vi "Get INFO from ini FILE - AMSServer.vi"(0 "ini Name":string="AMSServer.ini", 5 "Application Directory (Default if blank)":path, 11 "Error In":errorcluster) -> (1 "Settings":T3, 4 "ini Path":path=path "C:/Users/CK/workspace/LabVIEW/Configuration File Test/MyEXE.ini", 8 "AMS Connection Information":T1={"Connection "="SQL Server 32bit HPEnvy", "Username"="admin", "Password"="admin123"}, 10 "Settings Boolean":T2, 12 "MessageQ":string, 15 "Error Out":errorcluster)   [LabVIEW 2013]
uses:
  Controls/Connection Information Cluster.ctl
  <vilib>/Utility/config.llb/Read Key (String).vi
  <vilib>/Utility/config.llb/Read Key (Boolean).vi
  <vilib>/Utility/config.llb/NI_LVConfig.lvlib
  <vilib>/Utility/config.llb/Write Key (I32).vi
panel:
  out "Application Directory":path=path "C:/Users/CK/workspace/LabVIEW/Configuration File Test"
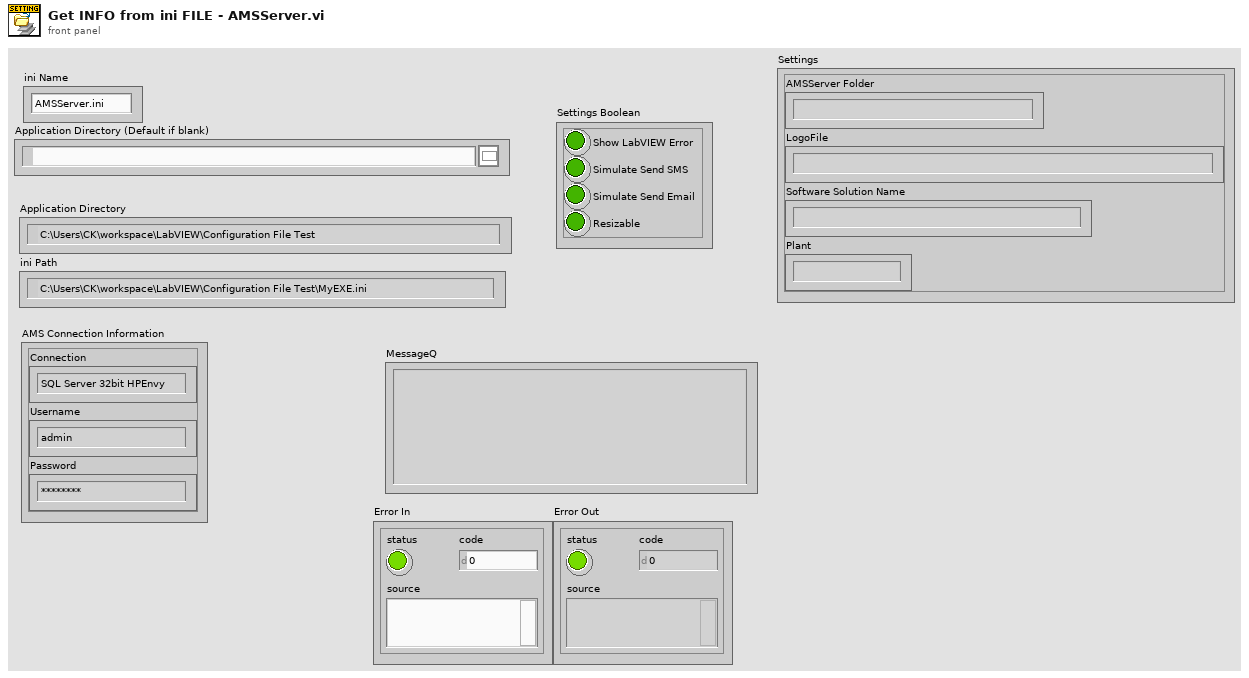
[diagram p1: front panel]
types:
  T1 = typedef "Connection Information Cluster.ctl" = cluster{"Connection ":string, "Username":string, "Password":string}
  T2 = cluster{"Show LabVIEW Error":bool, "Simulate Send SMS":bool, "Simulate Send Email":bool, "Resizable":bool}
  T3 = cluster{"AMSServer Folder":string, "LogoFile":string, "Software Solution Name":string, "Plant":string}
  T4 = typedef "NI_LVConfig.lvlib/Config Data RefNum.ctl" = refnum<k1>
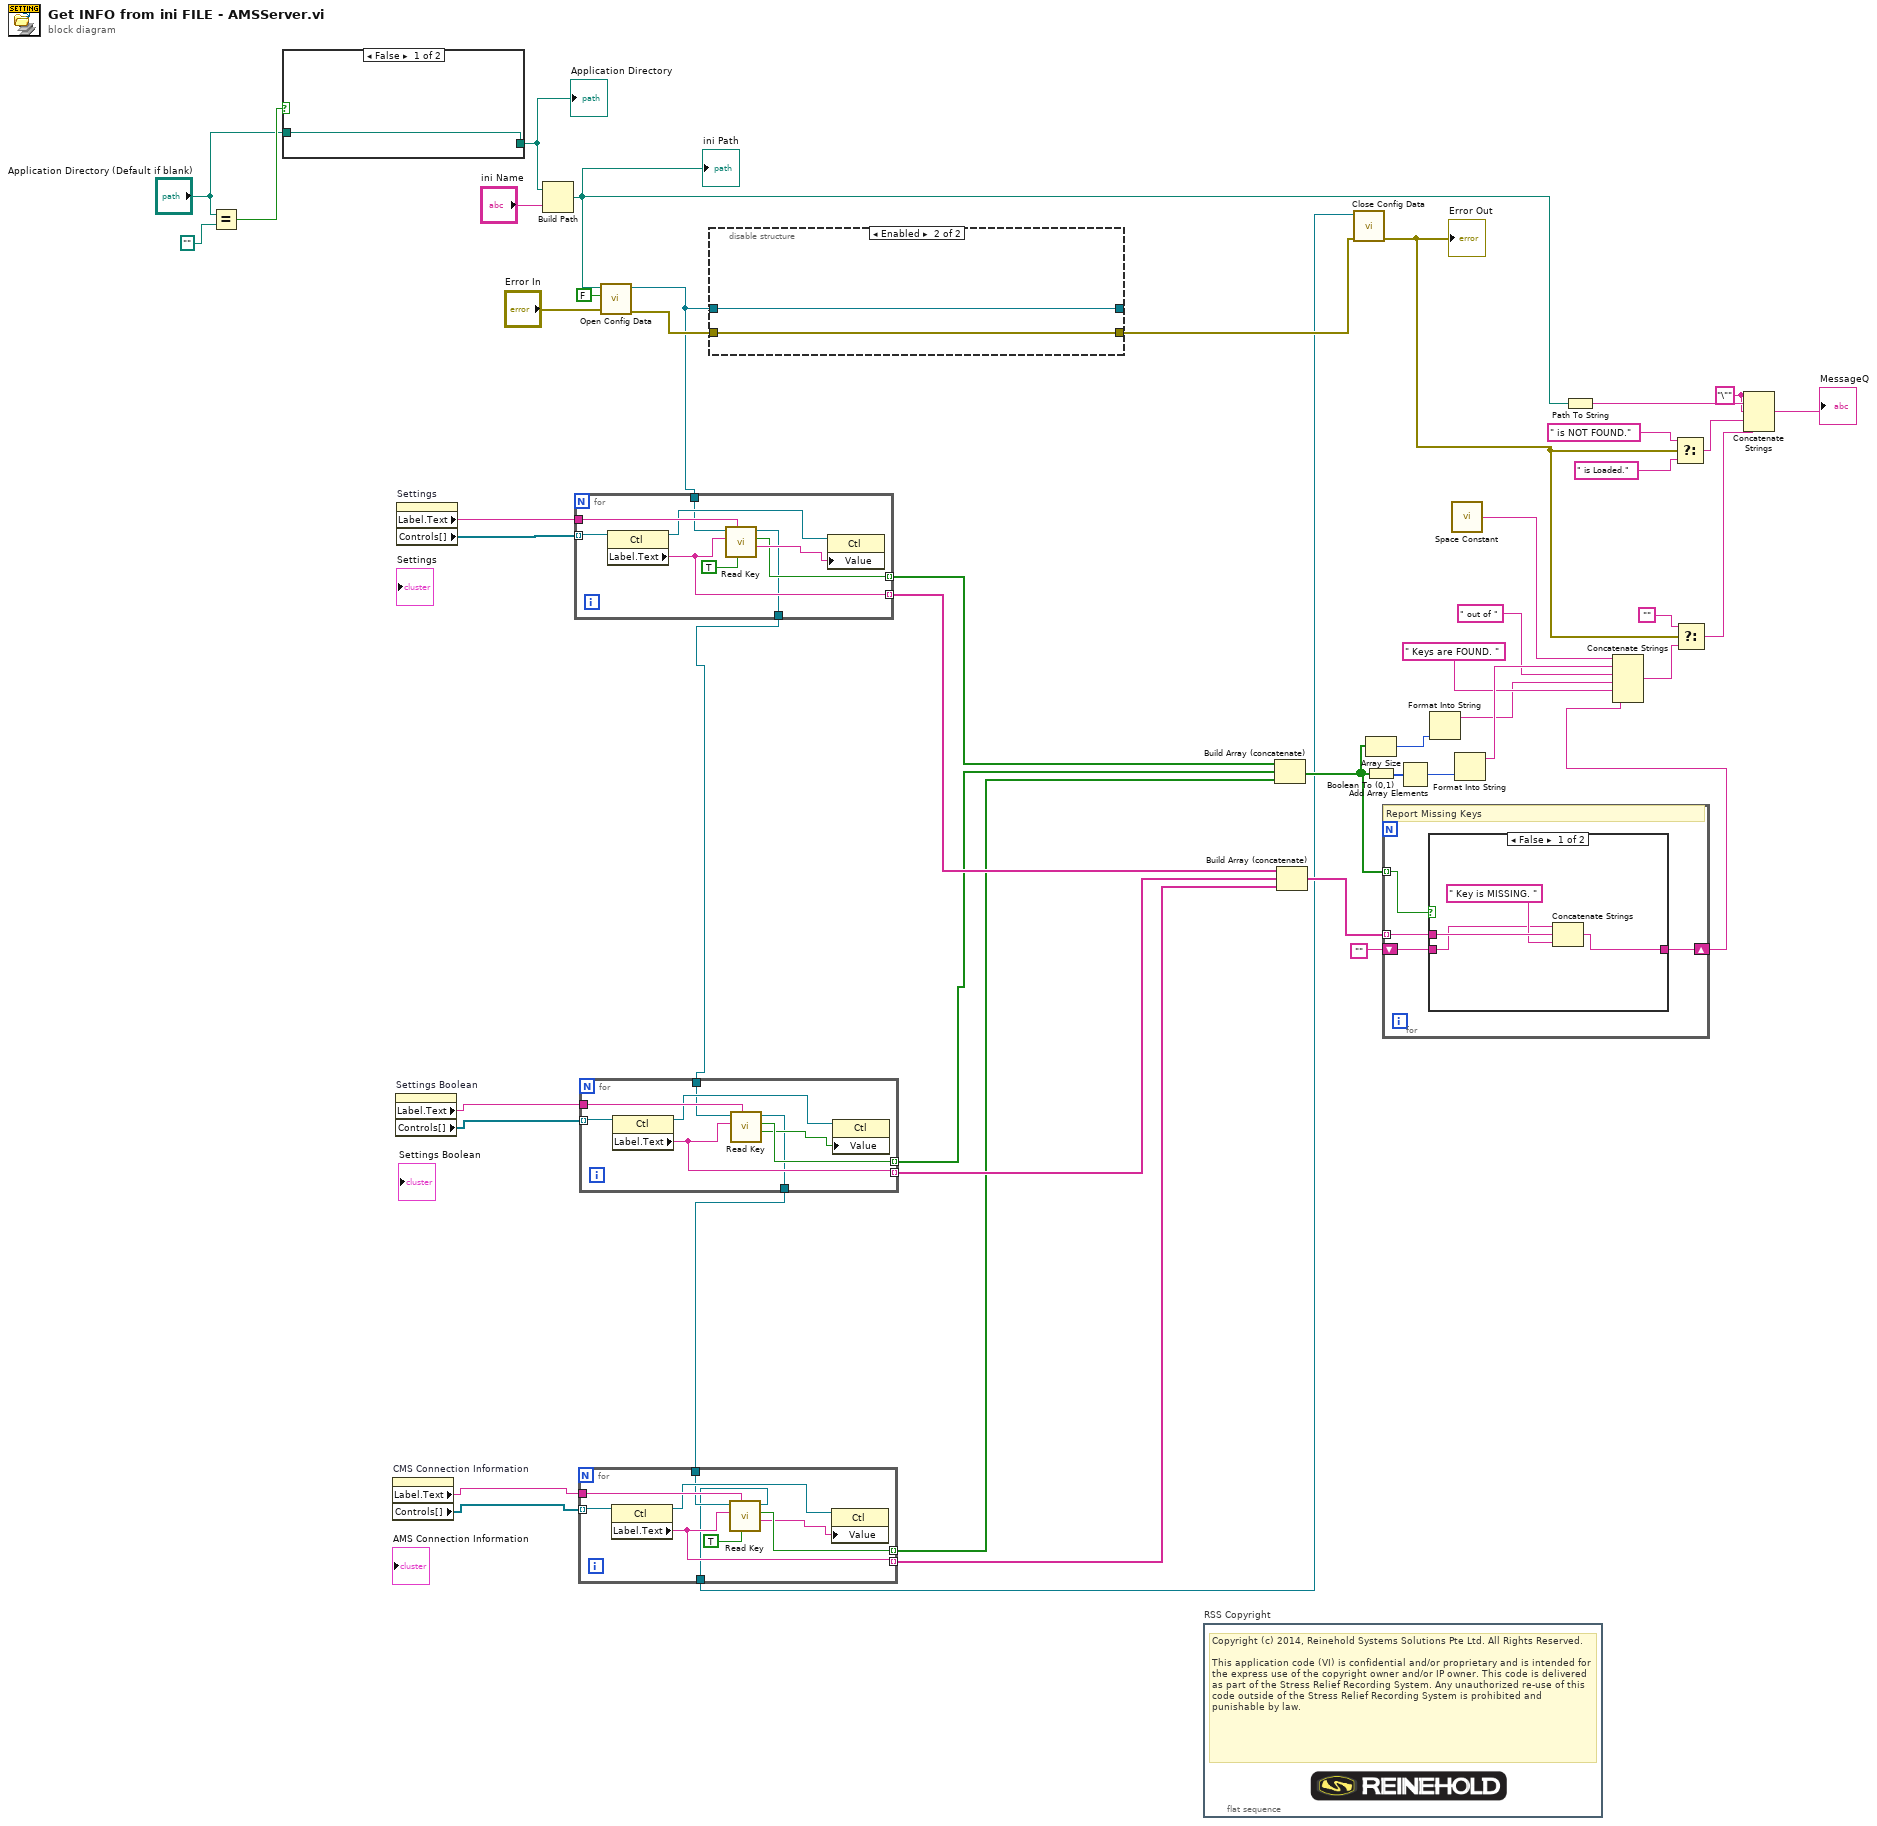
[diagram p0: block diagram]
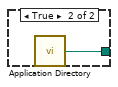
[diagram p2: hidden frame]
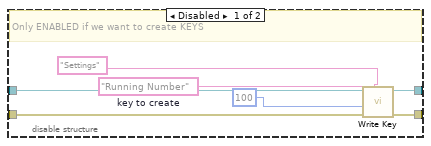
[diagram p4: hidden frame]
diagram:
  w42 = "\"" ("string")
  n1 = Equal?(x="Application Directory (Default if blank)", y=path "") -> (x = y?=w20:bool)
  n2 = case shown="False" w20 {
    tunnel: [w49 w50] -> w48
    tunnel: "Application Directory (Default if blank)" -> [w49 _]
    frame False {
    }
    frame True {
      n3 = call <vilib>:"Application Directory.vi"() -> ("Application Directory"=w50:path)
    }
  }
  "Application Directory" <- w48
  n4 = property on="CMS Connection Information" class="Clust (strict)"() -> ("Label.Text"=w6:string, "Controls[]"=w7:refnum<vi>[])  [unwired: 2 in, 2 out]
  n5 = property on="Settings Boolean" class="Clust (strict)"() -> ("Label.Text"=w8:string, "Controls[]"=w12:refnum<vi>[])  [unwired: 2 in, 2 out]
  n6 = property on="Settings" class="Clust (strict)"() -> ("Label.Text"=w16:string, "Controls[]"=w17:refnum<vi>[])  [unwired: 2 in, 2 out]
  n7 = Build Path(base path=w48, name or relative path="ini Name") -> (appended path=w44:path)
  "ini Path" <- w44
  n8 = call <vilib>:"Open Config Data.vi"("error in (no error)"="Error In", "create file if necessary (T)"=FALSE, "configuration file path"=w44) -> ("error out"=w45:errorcluster, "refnum"=w13:T4)  [unwired: 6 in, 1 out]
  n9 = for {
    tunnel: w17 -> [w59] mode=indexing
    tunnel: w16 -> [w58]
    tunnel: [w55] -> w15 mode=indexing
    tunnel: w13 -> [w54]
    tunnel: [w53] -> w14 mode=indexing
    tunnel: [w52] -> w2
    n10 = property class="Ctl"(reference=w59) -> (reference out=w57:refnum<vi>, "Label.Text"=w53:string)  [unwired: 1 in, 1 out]
    n11 = call-poly <vilib>:"Read Key.vi"("read raw string? (F)"=TRUE, "section"=w58, "key"=w53, "refnum"=w54) -> ("value"=w56:string, "found?"=w55:bool, "refnum out"=w52:T4)  [unwired: 4 in, 1 out]
    n12 = property class="Ctl"(reference=w57, "Value"=w56) -> ()  [unwired: 1 in, 2 out]
  }
  n13 = for {
    tunnel: w12 -> [w67] mode=indexing
    tunnel: w8 -> [w66]
    tunnel: [w64] -> w10 mode=indexing
    tunnel: w2 -> [w63]
    tunnel: [w62] -> w11 mode=indexing
    tunnel: [w60] -> w1
    n14 = property class="Ctl"(reference=w67) -> (reference out=w65:refnum<vi>, "Label.Text"=w62:string)  [unwired: 1 in, 1 out]
    n15 = call-poly <vilib>:"Read Key.vi"("section"=w66, "key"=w62, "refnum"=w63) -> ("value"=w61:bool, "found?"=w64:bool, "refnum out"=w60:T4)  [unwired: 5 in, 1 out]
    n16 = property class="Ctl"(reference=w65, "Value"=w61) -> ()  [unwired: 1 in, 2 out]
  }
  n17 = for {
    tunnel: w7 -> [w76] mode=indexing
    tunnel: w6 -> [w75]
    tunnel: [w73] -> w4 mode=indexing
    tunnel: w1 -> [w72]
    tunnel: [w71] -> w3 mode=indexing
    tunnel: [w69] -> w5
    n18 = property class="Ctl"(reference=w76) -> (reference out=w74:refnum<vi>, "Label.Text"=w71:string)  [unwired: 1 in, 1 out]
    n19 = call-poly <vilib>:"Read Key.vi"("read raw string? (F)"=TRUE, "section"=w75, "key"=w71, "refnum"=w72) -> ("value"=w70:string, "found?"=w73:bool, "refnum out"=w69:T4)  [unwired: 4 in, 1 out]
    n20 = property class="Ctl"(reference=w74, "Value"=w70) -> ()  [unwired: 1 in, 2 out]
  }
  n21 = disable-structure shown="Enabled" {
    disable-tunnel: w45 -> [w83 w84]
    disable-tunnel: [w80 w84] -> w9
    disable-tunnel: [w81 w85] -> _
    disable-tunnel: w13 -> [w82 w85]
    frame Disabled {
      w79 = "Running Number"  # key to create
      # "Only ENABLED if we want to create KEYS"
      n22 = call-poly <vilib>:"Write Key.vi"("section"="Settings", "error in (no error)"=w83, "value"=100 ("default value"), "key"=w79, "refnum"=w82) -> ("error out"=w80:errorcluster, "refnum out"=w81:T4)  [unwired: 4 in, 1 out]
    }
    frame Enabled {
    }
  }
  n23 = flat-sequence "RSS Copyright" {
    frame #0 {
      # "Copyright (c) 2014, Reinehold Systems Solutions Pte Ltd. All Rights Reserved.\n\nThis application code (VI) is confidential and/or proprietary and is intended for the express use of the copyright owner and/or IP owner. This code is delivered as part of the Stress Relief Recording System. Any unauthorized re-use of this code outside of the Stress Relief Recording System is prohibited and punishable by law."
    }
  }
  n24 = Build Array (concatenate)(w15, w10, w4) -> (w24:bool[])
  n25 = Build Array (concatenate)(w14, w11, w3) -> (w18:string[])
  n26 = call <vilib>:"Close Config Data.vi"("error in (no error)"=w9, "refnum"=w5) -> ("error out"=w28:errorcluster)  [unwired: 8 in, 1 out]
  "Error Out" <- w28
  n27 = Array Size(array=w24) -> (size(s)=w23:i32)
  n28 = Boolean To (0,1)(Boolean=w24) -> (0, 1=w37:i16[])
  n29 = for {
    tunnel: w24 -> [w89] mode=indexing
    tunnel: w18 -> [w88] mode=indexing
    shift-right: [w86] -> w26
    shift-left: "" -> [w87]
    # "Report Missing Keys"
    n30 = case shown="False" w89 {
      tunnel: w88 -> [w93 _]
      tunnel: w87 -> [w91 w94]
      tunnel: [w90 w94] -> w86
      frame False {
        n31 = Concatenate Strings(w91, w93, " Key is MISSING. " ("string")) -> (w90:string)
      }
      frame True {
      }
    }
  }
  n32 = Add Array Elements(numeric array=w37) -> (sum=w36:i16)
  n33 = Format Into String(w23) -> (resulting string=w22:string)  [unwired: 3 in, 1 out]
  n34 = call <vilib>:"Space Constant.vi"() -> ("String"=w34:string)
  n35 = Format Into String(w36) -> (resulting string=w33:string)  [unwired: 3 in, 1 out]
  n36 = Path To String(path=w44) -> (string=w43:string)
  n37 = Concatenate Strings(w34, w33, " out of " ("string"), w22, " Keys are FOUND. " ("string"), w26) -> (w31:string)
  n38 = Select(t=" is NOT FOUND." ("string"), s=w28, f=" is Loaded." ("string")) -> (s? t:f=w40:string)
  n39 = Select(t="", s=w28, f=w31) -> (s? t:f=w30:string)
  n40 = Concatenate Strings(w42, w43, w42, w40, w30) -> (→"MessageQ":string)
